vi "Pockels Cal-Objective cal confirm.vi"(11 "Index of current outer loop iteraton":i32) -> (0 "error out":errorcluster, 1 "Cancelled":bool, 2 "Skip cal for this objective":bool, 3 "Skip cal for all objectives":bool)   [LabVIEW 2013]
uses:
  Globals/gl_Calibration globals.vi
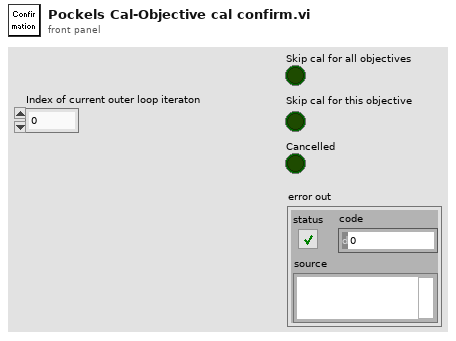
[diagram p1: front panel]
types:
  T1 = typedef "Pockels cal process refs.ctl" = cluster{"This VI":refnum<vi>, "Abort (ind)":refnum<vi>, "Next (ind)":refnum<vi>, "Cancel":refnum<vi>, "Next":refnum<vi>, "Message":refnum<vi>, "Measured Power ctrl":refnum<vi>, "Measured Power ind":refnum<vi>, "Pockels cal progress bar":refnum<vi>, "Abort this objective":refnum<vi>}
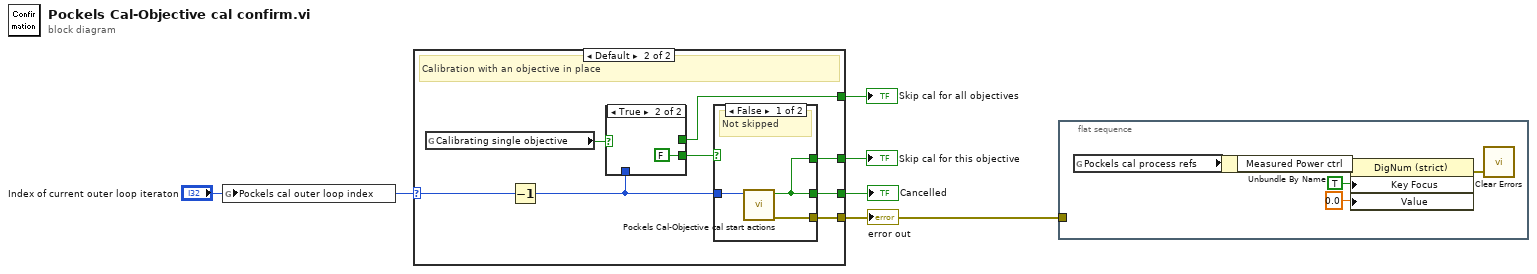
[diagram p0: block diagram]
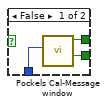
[diagram p3: hidden frame]
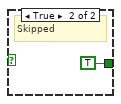
[diagram p4: hidden frame]
diagram:
  n1 = global write "gl_Calibration globals.vi" "Pockels cal outer loop index"("Index of current outer loop iteraton") -> ()
  n2 = case shown="Default" "Index of current outer loop iteraton" {
    selector: "Index of current outer loop iteraton" -> [_ w10]
    tunnel: [_ w13] -> w3
    tunnel: [_ w11] -> w5
    tunnel: [_ w9] -> w4
    tunnel: [_ w6] -> w1
    frame 0 {
      # "Calibration without an objective in place"
    }
    frame Default {
      # "Calibration with an objective in place"
      n3 = global read "gl_Calibration globals.vi" "Calibrating single objective"() -> (w7:bool)
      n4 = Decrement(x=w10) -> (x-1=w8:i32)
      n5 = case shown="True" w7 {
        tunnel: [w16 FALSE ("Cancelled (Left button pressed)")] -> w12
        tunnel: [w15 _] -> w9
        tunnel: w8 -> [w14 _]
        frame False {
          n6 = call "Pockels Cal-Message window.vi"("Objective index"=w14) -> ("Cancelled (Left button pressed)"=w16:bool, "Finish"=w15:bool)  [unwired: 8 in, 1 out]
        }
        frame True {
        }
      }
      n7 = case shown="False" w12 {
        tunnel: [w20 _] -> w13
        tunnel: w8 -> [w19 _]
        tunnel: [w18 TRUE] -> w11
        tunnel: [w18 _] -> w6
        frame False {
          # "Not skipped"
          n8 = call "Pockels Cal-Objective cal start actions.vi"("Objective index"=w19) -> ("error out"=w20:errorcluster, "Cancelled (Left button pressed)"=w18:bool)  [unwired: 9 in]
        }
        frame True {
          # "Skipped"
        }
      }
    }
  }
  "error out" <- w3
  "Skip cal for this objective" <- w5
  "Skip cal for all objectives" <- w4
  "Cancelled" <- w1
  n9 = flat-sequence {
    tunnel: w3 -> [_]
    frame #0 {
      n10 = global read "gl_Calibration globals.vi" "Pockels cal process refs"() -> (w24:T1)
      n11 = Unbundle By Name(w24) -> ("Measured Power ctrl"=w23:refnum<vi>)
      n12 = property on="Property Node" class="DigNum (strict)"(reference=w23, "Key Focus"=TRUE, "Value"=0.0 ("Measured Power")) -> (error out=w22:errorcluster)  [unwired: 1 in, 1 out]
      n13 = call <vilib>:"Clear Errors.vi"("error in (no error)"=w22) -> ()  [unwired: 6 in, 1 out]
    }
  }
